vi "Driver Get All.vi"(6 "Descending? (F)":bool, 8 "error in (no error)":errorcluster, 10 "Sort by (sxDriverId)":T2, 11 "Connection Refnum":T1) -> (0 "error out":errorcluster, 2 "Drivers":T3[](array[typedef]), 3 "Connection Refnum":T1, 4 "Data Present?":bool)   [LabVIEW 2011]
uses:
  Driver Record.ctl
  Driver Table Fields.ctl
  SI.LIB/ODBC/SQL Controls/Connection Refnum.ctl
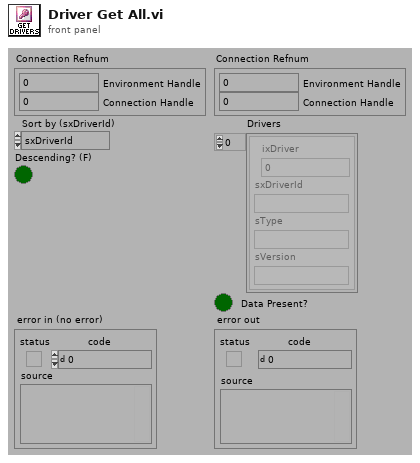
[diagram p1: front panel]
types:
  T1 = typedef "Connection Refnum.ctl" = cluster{"Environment Handle":i32, "Connection Handle":i32}
  T2 = typedef "Driver Table Fields.ctl" = enum16{"sxDriverId", "sType", "sVersion", "ixDriver"}
  T3 = typedef "Driver Record.ctl" = cluster{"ixDriver":i32, "sxDriverId":string, "sType":string, "sVersion":string}
  T4 = typedef "Statement Refnum.ctl" = cluster{"Statement Handle":i32, "Parameter Number":u16}
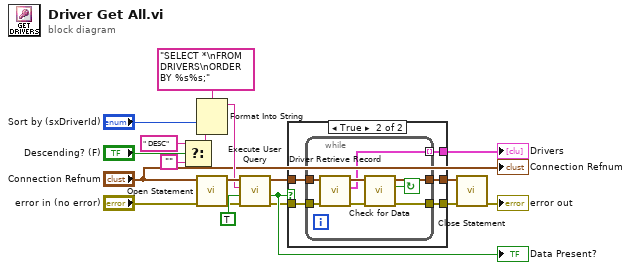
[diagram p0: block diagram]
diagram:
  n1 = Select(t=" DESC" ("input 2"), s="Descending? (F)", f="") -> (s? t:f=w5:string)
  n2 = Format Into String(format string="SELECT *\nFROM DRIVERS\nORDER BY %s%s;" ("Query Name"), "Sort by (sxDriverId)", w5) -> (resulting string=w11:string)  [unwired: 2 in, 1 out]
  n3 = call "Open Statement.vi"("error in (no error)"="error in (no error)", "Connection Refnum"="Connection Refnum") -> ("error out"=w14:errorcluster, "Statement Refnum"=w15:T4)  [unwired: 4 out]
  n4 = call "Execute User Query.vi"("error in (no error)"=w14, "Return Data? (f)"=TRUE, "User Query"=w11, "Statement Refnum"=w15) -> ("error out"=w18:errorcluster, "Data Present?"=w19:bool, "Statement Refnum"=w17:T4)  [unwired: 1 out]
  "Data Present?" <- w19
  n5 = case shown="True" w19 {
    tunnel: w18 -> [w20 w26]
    tunnel: w17 -> [w21 w25]
    tunnel: [w20 w24] -> w13
    tunnel: [w21 w23] -> w12
    tunnel: [_ w22] -> w3
    frame False {
    }
    frame True {
      n6 = while {
        tunnel: w26 -> [w31]
        tunnel: w25 -> [w30]
        tunnel: [w33] -> w24
        tunnel: [w32] -> w23
        tunnel: [w27] -> w22 mode=indexing
        stop <- w34 continue-if-true
        n7 = call "Driver Retrieve Record.vi"("error in (no error)"=w31, "Statement Refnum"=w30) -> ("error out"=w28:errorcluster, "Driver Record"=w27:T3, "Statement Refnum"=w29:T4)  [unwired: 7 out]
        n8 = call "Check for Data.vi"("error in (no error)"=w28, "Statement Refnum"=w29) -> ("error out"=w33:errorcluster, "Data Present?"=w34:bool, "Statement Refnum"=w32:T4)  [unwired: 3 out]
      }
    }
  }
  "Drivers" <- w3
  n9 = call "Close Statement.vi"("error in (no error)"=w13, "Statement Refnum"=w12) -> ("error out"=→"error out":errorcluster)  [unwired: 5 out]
  "Connection Refnum" <- "Connection Refnum"
